vi "get_STM_Status_string (SubVI).vi"(8 "error in (no error)":errorcluster, 11 "Application in":refnum<vi>) -> (0 "error out":errorcluster, 2 "JSON string":string, 3 "Application out":refnum<vi>)   [LabVIEW 2014]
uses:
  <userlib>/Nanonis Prog Interface V5/Nanonis Prog Interface.lvlib
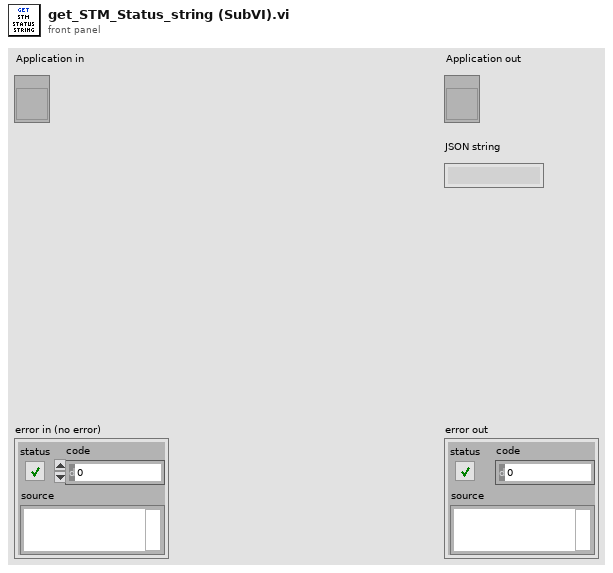
[diagram p1: front panel]
types:
  T1 = cluster{"Center coordinates (m)":cluster{"Xc":sgl, "Yc":sgl}, "Z position (m)":sgl, "Current (A)":sgl, "Size (m)":cluster{"Width":sgl, "Height":sgl}}
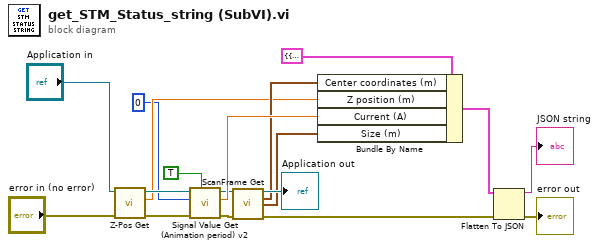
[diagram p0: block diagram]
diagram:
  n1 = call <userlib>:"Z-Pos Get.vi"("error in (no error)"="error in (no error)", "Application ref in"="Application in") -> ("error out"=w12:errorcluster, "Z position (m)"=w6:sgl, "Application ref out"=w9:refnum<vi>)  [unwired: 7 in]
  n2 = call <userlib>:"Signal Value Get (Animation period) v2.vi"("Wait for newest data (F=False)"=TRUE, "error in (no error)"=w12, "Signal index (0-79)"=i8 0, "Application ref in"=w9) -> ("error out"=w11:errorcluster, "Signal value"=w14:sgl, "Application ref out"=w10:refnum<vi>)  [unwired: 4 in]
  n3 = call <userlib>:"ScanFrame Get.vi"("Application ref in"=w10, "error in (no error)"=w11) -> ("Application ref out"=→"Application out":refnum<vi>, "Center coordinates (m)"=w7:cluster{"Xc":sgl, "Yc":sgl}, "Size (m)"=w8:cluster{"Width":sgl, "Height":sgl}, "error out"=w2:errorcluster)  [unwired: 9 in, 1 out]
  n4 = Bundle By Name(cluster=T1 {"Center coordinates (m)"={"Xc"=0.0, "Yc"=0.0}, "Z position (m)"=0.0, "Current (A)"=0.0, "Size (m)"={"Width"=0.0, "Height"=0.0}} ("STMStatus"), "Center coordinates (m)"=w7, "Z position (m)"=w6, "Current (A)"=w14, "Size (m)"=w8) -> (w5:T1)
  n5 = Flatten To JSON(anything=w5, error in (no error)=w2) -> (JSON string=→"JSON string":string, 11:→"error out":errorcluster)  [unwired: 1 in]
